vi "Main.vi"() -> ()   [LabVIEW 2017]
doc: "The myRIO Project template acquires acceleration data from the onboard accelerometer and displays the changes of acceleration values in a waveform chart."
uses:
  <vilib>/myRIO/Common/Instrument Driver Framework/myRIO v1.0/Encoder/typedefs/Encoder Count Direction Enum.ctl
  Motor Status Enum.ctl
  <vilib>/myRIO/Instrument Drivers/Onboard IO/PWM/typedefs/PWM Reference.ctl
  <vilib>/myRIO/Common/Instrument Driver Framework/Utilities/typedefs/myRIO Generic Hardware Reference.ctl
  <vilib>/myRIO/Common/Instrument Driver Framework/Utilities/typedefs/Hardware Version Enum.ctl
  <vilib>/myRIO/Common/Instrument Driver Framework/Utilities/typedefs/myRIO v1.0 Reference.ctl
  <vilib>/myRIO/Common/Instrument Driver Framework/Utilities/typedefs/Generic FPGA Reference.ctl
  <vilib>/myRIO/Common/Instrument Driver Framework/myRIO v1.0/PWM/typedefs/PWM Channels Enum.ctl
  <vilib>/myRIO/Instrument Drivers/Onboard IO/PWM/typedefs/PWM Configuration.ctl
  <vilib>/userdefined/High Color/nirio_resource_hc.ctl
  <vilib>/myRIO/Common/Instrument Driver Framework/Utilities/vis/Is FPGA Ref Available.vi
  <vilib>/myRIO/Common/Instrument Driver Framework/myRIO v1.0/PWM/vis/myRIO v1.1 Open PWM.vi
  <vilib>/myRIO/Instrument Drivers/Onboard IO/PWM/vis/Set Duty Cycle and Frequency.vi
  <vilib>/myRIO/Common/Instrument Driver Framework/Utilities/vis/Validate Channels.vi
  <vilib>/myRIO/Common/Instrument Driver Framework/myRIO v1.0/PWM/vis/myRIO v1.0 Reserve PWM.vi
  <vilib>/myRIO/Common/Instrument Driver Framework/myRIO v1.0/UART/vis/myRIO v1.0 Close UART.vi
  <vilib>/myRIO/Common/Instrument Driver Framework/myRIO v1.0/PWM/vis/myRIO v1.0 Build MUX Configuration PWM.vi
  <vilib>/myRIO/Common/Instrument Driver Framework/myRIO v1.0/Resource Manager/vis/myRIO v1.0 Reserve Channel List.vi
  <vilib>/myRIO/Common/Instrument Driver Framework/myRIO v1.0/Resource Manager/vis/myRIO v1.0 Create Configuration List.vi
  <vilib>/myRIO/Common/Instrument Driver Framework/myRIO v1.0/Resource Manager/vis/myRIO v1.0 Reserve Channel.vi
  <vilib>/myRIO/Common/Instrument Driver Framework/myRIO v1.0/Resource Manager/vis/myRIO v1.0 Unreserve Channel.vi
  <vilib>/myRIO/Common/Instrument Driver Framework/myRIO v1.0/Resource Manager/vis/myRIO v1.0 Build Mutex Name.vi
  <vilib>/Utility/VariantDataType/GetNumericInfo.vi
  <vilib>/Utility/error.llb/Error Cluster From Error Code.vi
  <vilib>/myRIO/Common/Instrument Driver Framework/myRIO v1.0/myRIO v1.1 Open.vi
  <vilib>/myRIO/Common/Instrument Driver Framework/Utilities/vis/IO Manager.vi
  <vilib>/myRIO/Common/Instrument Driver Framework/Utilities/vis/Configuration Manager.vi
  <vilib>/myRIO/Common/Instrument Driver Framework/myRIO v1.0/Resource Manager/vis/myRIO v1.0 Configure IO.vi
  <vilib>/myRIO/Common/Instrument Driver Framework/myRIO v1.0/myRIO v1.0 Close.vi
  <vilib>/myRIO/Common/Instrument Driver Framework/myRIO v1.0/PWM/vis/myRIO v1.0 Write PWM.vi
  <vilib>/myRIO/Common/Instrument Driver Framework/Utilities/vis/FPGA Ref Manager.vi
  <vilib>/myRIO/Common/Instrument Driver Framework/myRIO v1.0/myRIO v1.0 Reset FPGA.vi
  <vilib>/myRIO/Common/Instrument Driver Framework/myRIO v1.0/IRQ/vis/myRIO v1.0 IRQ Info FGV.vi
  <vilib>/myRIO/Common/Instrument Driver Framework/myRIO v1.0/IRQ/vis/myRIO v1.0 Timer IRQ Info FGV.vi
  <vilib>/myRIO/Common/Instrument Driver Framework/myRIO v1.0/IRQ/vis/myRIO v1.0 ISR Agent.vi
  <vilib>/myRIO/Express VI/Onboard IO/PWM/PWM Express VI.xnode
  <vilib>/myRIO/Instrument Drivers/Onboard IO/PWM/vis/myRIO PWM Open.xnode
  <vilib>/myRIO/Instrument Drivers/Utilities/Utilities.lvlib
  <vilib>/myRIO/Instrument Drivers/Onboard IO/PWM/PWM.lvlib
panel:
  out "X Axis state":T1
  out "Y Axis state":T1
  out "Loop Runtime (s)":u32
  in  "Clear Chart History":bool
  in  "Coordinates Input":cluster{"X-axis (mm)":dbl, "Y-axis (mm)":dbl}
  out "Y Axis":T2(graph)
  out "X Axis":T2(graph)
  in  "X Axis Motor Target":T3
  out "X Axis Motor Params":T4
  in  "Y Axis Motor Target":T5
  out "Y Axis Motor Params":T5
  in  "stop":bool
  out "Output String":string
  out "Encoder Output":T7
  out "Total Runtime (s)":dbl format="%.2f"
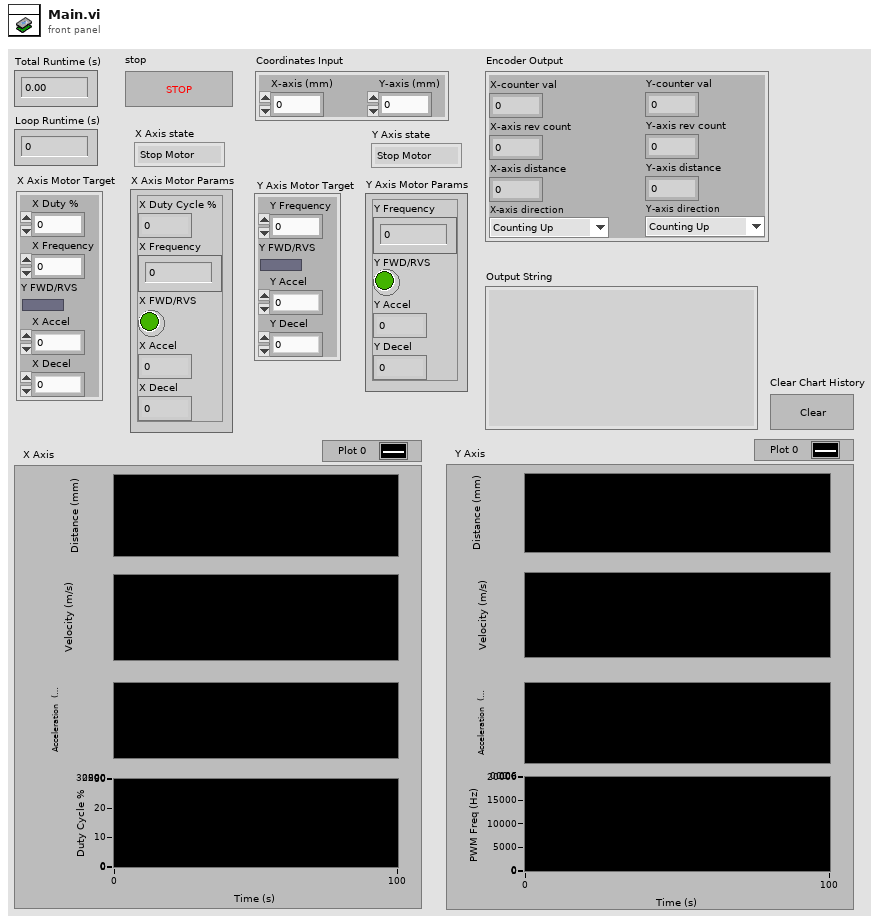
[diagram p1: front panel]
types:
  T1 = typedef "Motor Status Enum.ctl" = enum16{"Stop Motor", "Read Inputs", "Steady Speed", "Accelerate", "Decelerate"}
  T2 = cluster{"X-axis distance":dbl, dbl, dbl, "X Frequency":dbl}
  T3 = cluster{"X Frequency":dbl, "Y FWD/RVS":bool, "X Accel":dbl, "X Decel":dbl, "X Duty %":dbl}
  T4 = cluster{"X Frequency":dbl, "X FWD/RVS":bool, "X Accel":dbl, "X Decel":dbl, "X Duty Cycle %":dbl}
  T5 = cluster{"Y Frequency":dbl, "Y FWD/RVS":bool, "Y Accel":dbl, "Y Decel":dbl}
  T6 = typedef "Encoder Count Direction Enum.ctl" = enum16{"Counting Up", "Counting Down"}
  T7 = cluster{"Y-axis rev count":dbl, "Y-axis distance":dbl, "X-axis rev count":dbl, "X-axis distance":dbl, "Y-axis direction":T6, "X-axis direction":T6, "X-counter val":i32, "Y-counter val":i32}
  T8 = cluster{"X-axis distance":dbl, dbl, dbl, "X Frequency":dbl}[]
  T9 = cluster{dbl, dbl, "X-axis distance":dbl, "X Duty Cycle %":dbl, "X Frequency":dbl, "Y-axis distance":dbl, "Y Frequency":dbl, "X Accel":dbl, "X Decel":dbl, "Y Accel":dbl, "Y Decel":dbl, "X-axis (mm)":dbl, "Y-axis (mm)":dbl}
  T10 = cluster{"X-axis distance":dbl, dbl, dbl, "X Duty Cycle %":dbl}
  T11 = cluster{"Y-axis distance":dbl, dbl, dbl, "Y Frequency":dbl}
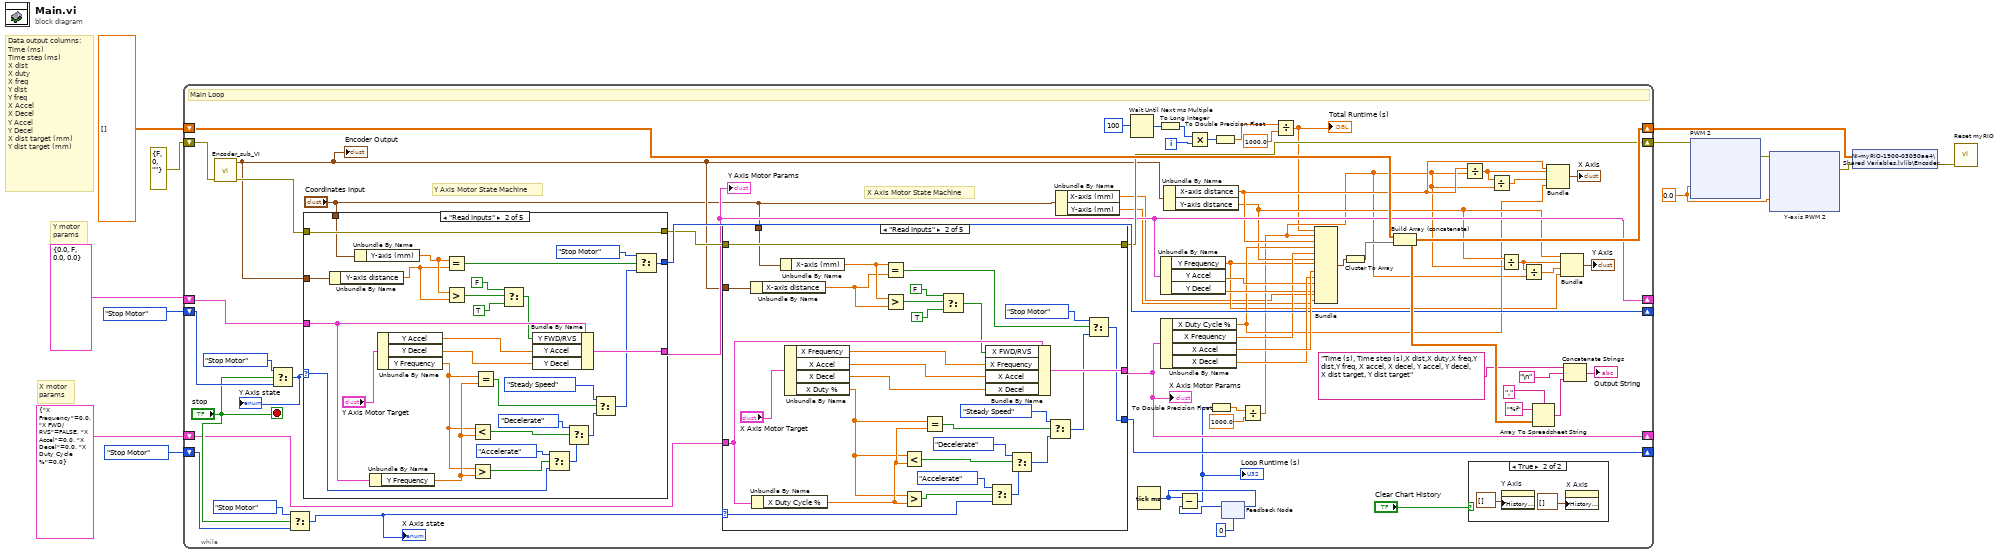
[diagram p0: block diagram]
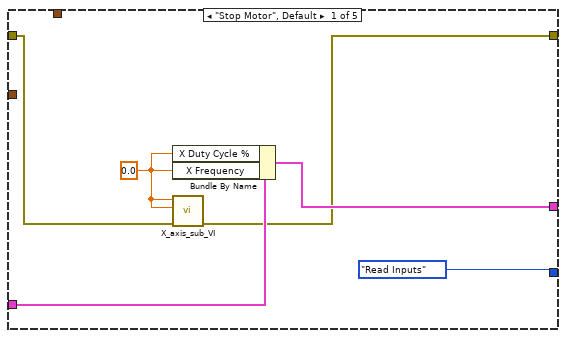
[diagram p3: hidden frame]
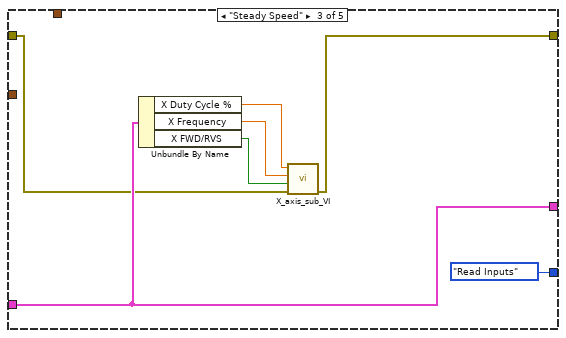
[diagram p4: hidden frame]
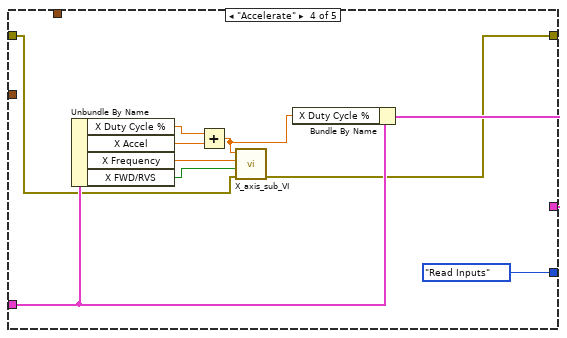
[diagram p5: hidden frame]
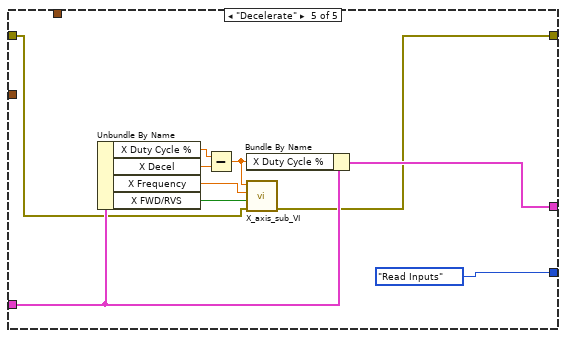
[diagram p6: hidden frame]
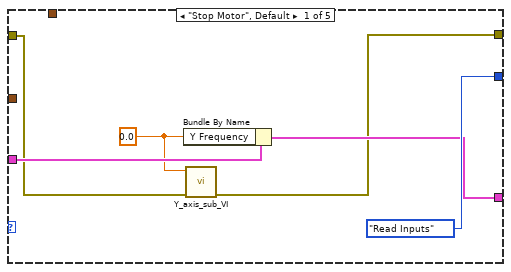
[diagram p7: hidden frame]
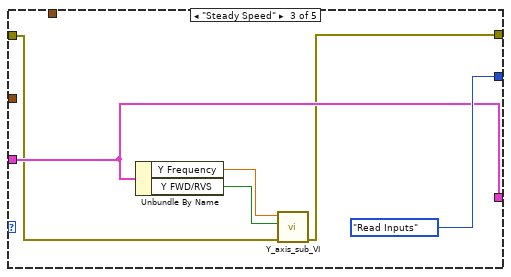
[diagram p8: hidden frame]
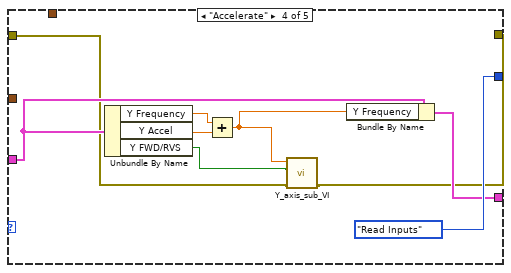
[diagram p9: hidden frame]
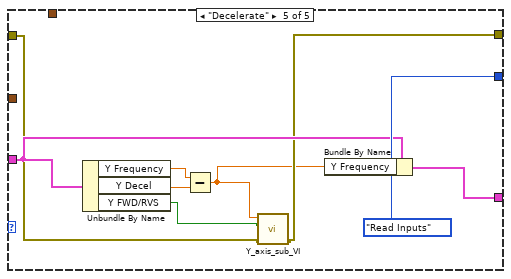
[diagram p10: hidden frame]
diagram:
  w5 = 0.0 ("Frequency [Hz]")
  # "X motor \nparams"
  # "Y motor \nparams"
  # "Data output columns:\nTime (ms)\nTime step (ms)\nX dist\nX duty\nX freq\nY dist\nY freq\nX Accel\nX Decel\nY Accel\nY Decel\nX dist target (mm)\nY dist target (mm)"
  n1 = while {
    shift-right: [w47] -> w12
    shift-left: errorcluster {"status"=FALSE, "code"=0, "source"=""} ("error in (no error)") -> [w74]
    shift-right: [w70] -> w8
    shift-left: dbl[][] [] -> [w69]
    shift-right: [w39] -> _
    shift-left: T5 {"Y Frequency"=0.0, "Y FWD/RVS"=FALSE, "Y Accel"=0.0, "Y Decel"=0.0} ("Y Axis Motor Params 2") -> [w60]
    shift-right: [w59] -> _
    shift-left: Motor_Status_Enum."Stop Motor" -> [w57]
    shift-right: [w50] -> _
    shift-left: Motor_Status_Enum."Stop Motor" -> [w52]
    shift-right: [w40] -> _
    shift-left: T4 {"X Frequency"=0.0, "X FWD/RVS"=FALSE, "X Accel"=0.0, "X Decel"=0.0, "X Duty Cycle %"=0.0} ("X Axis Motor Params 3") -> [w49]
    i -> [w73]
    stop <- "stop" stop-if-true
    # "X Axis Motor State Machine"
    # "Y Axis Motor State Machine"
    # "Main Loop"
    n2 = call "Encoder_sub_VI.vi"("error in (no error)"=w74) -> ("error out"=w55:errorcluster, "Encoder Output"=w38:T7)  [unwired: 9 in]
    "Encoder Output" <- w38
    n3 = Select(t=Motor_Status_Enum."Stop Motor", s="stop", f=w57) -> (s? t:f=w58:T1)
    "Y Axis state" <- w58
    n4 = Select(t=Motor_Status_Enum."Stop Motor", s="stop", f=w52) -> (s? t:f=w53:T1)
    "X Axis state" <- w53
    n5 = case shown="\"Read Inputs\"" w58 {
      selector: w58 -> [_ w160 _ _ _]
      tunnel: w60 -> [w145 w161 w177 w186 w194]
      tunnel: [Motor_Status_Enum."Read Inputs" w152 Motor_Status_Enum."Read Inputs" Motor_Status_Enum."Read Inputs" Motor_Status_Enum."Read Inputs"] -> w59
      tunnel: [w143 w162 w177 w185 w195] -> w39
      tunnel: w55 -> [w141 w159 w176 w182 w192]
      tunnel: [w142 w159 w175 w181 w193] -> w48
      tunnel: w38 -> [_ w158 _ _ _]
      tunnel: "Coordinates Input" -> [_ w146 _ _ _]
      frame "Stop Motor", Default {
        w140 = 0.0 ("Y Frequency")
        n6 = Bundle By Name(cluster=w145, "Y Frequency"=w140) -> (w143:T5)
        n7 = call "Y_axis_sub_VI.vi"("error in (no error)"=w141, "Frequency"=w140) -> ("error out"=w142:errorcluster)  [unwired: 9 in]
      }
      frame "Read Inputs" {
        n8 = Unbundle By Name(w158) -> ("Y-axis distance"=w155:dbl)
        n9 = Unbundle By Name(w146) -> ("Y-axis (mm)"=w156:dbl)
        n10 = Unbundle By Name(w161) -> ("Y Frequency"=w168:dbl)
        n11 = Unbundle By Name("Y Axis Motor Target") -> ("Y Accel"=w172:dbl, "Y Decel"=w173:dbl, "Y Frequency"=w157:dbl)
        n12 = Equal?(x=w156, y=w155) -> (x = y?=w154:bool)
        n13 = Greater?(x=w156, y=w155) -> (0:w150:bool)
        n14 = Less?(x=w157, y=w168) -> (x < y?=w165:bool)
        n15 = Greater?(x=w157, y=w168) -> (0:w174:bool)
        n16 = Equal?(x=w157, y=w168) -> (x = y?=w169:bool)
        n17 = Select(t=FALSE, s=w150, f=TRUE) -> (s? t:f=w147:bool)
        n18 = Bundle By Name(cluster=w161, "Y FWD/RVS"=w147, "Y Accel"=w172, "Y Decel"=w173) -> (w162:T5)
        n19 = Select(t=Motor_Status_Enum."Accelerate", s=w174, f=w160) -> (s? t:f=w167:T1)
        n20 = Select(t=Motor_Status_Enum."Decelerate", s=w165, f=w167) -> (s? t:f=w170:T1)
        n21 = Select(t=Motor_Status_Enum."Steady Speed", s=w169, f=w170) -> (s? t:f=w151:T1)
        n22 = Select(t=Motor_Status_Enum."Stop Motor", s=w154, f=w151) -> (s? t:f=w152:T1)
      }
      frame "Steady Speed" {
        n23 = Unbundle By Name(w177) -> ("Y Frequency"=w179:dbl, "Y FWD/RVS"=w180:bool)
        n24 = call "Y_axis_sub_VI.vi"("error in (no error)"=w176, "FWD/RVS"=w180, "Frequency"=w179) -> ("error out"=w175:errorcluster)  [unwired: 8 in]
      }
      frame "Accelerate" {
        n25 = Unbundle By Name(w186) -> ("Y Frequency"=w188:dbl, "Y Accel"=w189:dbl, "Y FWD/RVS"=w183:bool)
        n26 = Add(x=w188, y=w189) -> (x+y=w184:dbl)
        n27 = call "Y_axis_sub_VI.vi"("error in (no error)"=w182, "FWD/RVS"=w183, "Frequency"=w184) -> ("error out"=w181:errorcluster)  [unwired: 8 in]
        n28 = Bundle By Name(cluster=w186, "Y Frequency"=w184) -> (w185:T5)
      }
      frame "Decelerate" {
        n29 = Unbundle By Name(w194) -> ("Y Frequency"=w198:dbl, "Y Decel"=w197:dbl, "Y FWD/RVS"=w191:bool)
        n30 = Subtract(x=w198, y=w197) -> (x-y=w190:dbl)
        n31 = call "Y_axis_sub_VI.vi"("error in (no error)"=w192, "FWD/RVS"=w191, "Frequency"=w190) -> ("error out"=w193:errorcluster)  [unwired: 8 in]
        n32 = Bundle By Name(cluster=w194, "Y Frequency"=w190) -> (w195:T5)
      }
    }
    "Y Axis Motor Params" <- w39
    n33 = case shown="\"Read Inputs\"" w53 {
      selector: w53 -> [_ w100 _ _ _]
      tunnel: [Motor_Status_Enum."Read Inputs" w84 Motor_Status_Enum."Read Inputs" Motor_Status_Enum."Read Inputs" Motor_Status_Enum."Read Inputs"] -> w50
      tunnel: [w79 w99 w116 w123 w133] -> w40
      tunnel: w49 -> [w80 w98 w116 w122 w132]
      tunnel: w48 -> [w78 w96 w114 w121 w131]
      tunnel: [w77 w96 w113 w120 w130] -> w47
      tunnel: w38 -> [_ w94 _ _ _]
      tunnel: "Coordinates Input" -> [_ w83 _ _ _]
      frame "Stop Motor", Default {
        w82 = 0.0 ("Y Frequency")
        n34 = Bundle By Name(cluster=w80, "X Duty Cycle %"=w82, "X Frequency"=w82) -> (w79:T4)
        n35 = call "X_axis_sub_VI.vi"("error in (no error)"=w78, "Frequency"=w82, "Duty Cycle %"=w82) -> ("error out"=w77:errorcluster)  [unwired: 8 in]
      }
      frame "Read Inputs" {
        n36 = Unbundle By Name(w94) -> ("X-axis distance"=w89:dbl)
        n37 = Unbundle By Name(w98) -> ("X Duty Cycle %"=w111:dbl)
        n38 = Unbundle By Name(w83) -> ("X-axis (mm)"=w90:dbl)
        n39 = Unbundle By Name("X Axis Motor Target") -> ("X Frequency"=w103:dbl, "X Accel"=w101:dbl, "X Decel"=w102:dbl, "X Duty %"=w95:dbl)
        n40 = Equal?(x=w90, y=w89) -> (x = y?=w88:bool)
        n41 = Greater?(x=w90, y=w89) -> (0:w92:bool)
        n42 = Less?(x=w95, y=w111) -> (x < y?=w106:bool)
        n43 = Greater?(x=w95, y=w111) -> (0:w104:bool)
        n44 = Equal?(x=w95, y=w111) -> (x = y?=w110:bool)
        n45 = Select(t=FALSE, s=w92, f=TRUE) -> (s? t:f=w85:bool)
        n46 = Bundle By Name(cluster=w98, "X FWD/RVS"=w85, "X Frequency"=w103, "X Accel"=w101, "X Decel"=w102) -> (w99:T4)
        n47 = Select(t=Motor_Status_Enum."Accelerate", s=w104, f=w100) -> (s? t:f=w108:T1)
        n48 = Select(t=Motor_Status_Enum."Decelerate", s=w106, f=w108) -> (s? t:f=w109:T1)
        n49 = Select(t=Motor_Status_Enum."Steady Speed", s=w110, f=w109) -> (s? t:f=w86:T1)
        n50 = Select(t=Motor_Status_Enum."Stop Motor", s=w88, f=w86) -> (s? t:f=w84:T1)
      }
      frame "Steady Speed" {
        n51 = Unbundle By Name(w116) -> ("X Duty Cycle %"=w118:dbl, "X Frequency"=w117:dbl, "X FWD/RVS"=w119:bool)
        n52 = call "X_axis_sub_VI.vi"("error in (no error)"=w114, "FWD/RVS"=w119, "Frequency"=w117, "Duty Cycle %"=w118) -> ("error out"=w113:errorcluster)  [unwired: 7 in]
      }
      frame "Accelerate" {
        n53 = Unbundle By Name(w122) -> ("X Duty Cycle %"=w125:dbl, "X Accel"=w126:dbl, "X Frequency"=w127:dbl, "X FWD/RVS"=w129:bool)
        n54 = Add(x=w125, y=w126) -> (x+y=w128:dbl)
        n55 = call "X_axis_sub_VI.vi"("error in (no error)"=w121, "FWD/RVS"=w129, "Frequency"=w127, "Duty Cycle %"=w128) -> ("error out"=w120:errorcluster)  [unwired: 7 in]
        n56 = Bundle By Name(cluster=w122, "X Duty Cycle %"=w128) -> (w123:T4)
      }
      frame "Decelerate" {
        n57 = Unbundle By Name(w132) -> ("X Duty Cycle %"=w135:dbl, "X Decel"=w136:dbl, "X Frequency"=w137:dbl, "X FWD/RVS"=w139:bool)
        n58 = Subtract(x=w135, y=w136) -> (x-y=w138:dbl)
        n59 = Bundle By Name(cluster=w132, "X Duty Cycle %"=w138) -> (w133:T4)
        n60 = call "X_axis_sub_VI.vi"("error in (no error)"=w131, "FWD/RVS"=w139, "Frequency"=w137, "Duty Cycle %"=w138) -> ("error out"=w130:errorcluster)  [unwired: 7 in]
      }
    }
    "X Axis Motor Params" <- w40
    n61 = Unbundle By Name("Coordinates Input") -> ("X-axis (mm)"=w15:dbl, "Y-axis (mm)"=w14:dbl)
    n62 = Wait Until Next ms Multiple(millisecond multiple=u32 100 ("milliseconds to wait")) -> (millisecond timer value=w61:u32)
    n63 = Tick Count (ms)() -> (millisecond timer value=w23:u32)
    n64 = To Long Integer(number=w61) -> (32bit integer=w64:i32)
    n65 = Unbundle By Name(w39) -> ("Y Frequency"=w27:dbl, "Y Accel"=w66:dbl, "Y Decel"=w65:dbl)
    n66 = Unbundle By Name(w40) -> ("X Duty Cycle %"=w28:dbl, "X Frequency"=w33:dbl, "X Accel"=w68:dbl, "X Decel"=w67:dbl)
    n67 = Unbundle By Name(w38) -> ("X-axis distance"=w37:dbl, "Y-axis distance"=w31:dbl)
    n68 = Multiply(x=w64, y=w73) -> (x*y=w62:i32)
    n69 = To Double Precision Float(number=w62) -> (double precision float=w17:dbl)
    n70 = feedback-in #1(w23) -> ()
    n71 = feedback #1(u32 0) -> (w24:u32)
    n72 = Subtract(x=w23, y=w24) -> (x-y=w22:u32)
    "Loop Runtime (s)" <- w22
    n73 = To Double Precision Float(number=w22) -> (double precision float=w20:dbl)
    n74 = Divide(x=w20, y=1000.0) -> (x/y=w19:dbl)
    n75 = Divide(x=w17, y=1000.0) -> (x/y=w13:dbl)
    "Total Runtime (s)" <- w13
    n76 = Bundle(w13, w19, "X-axis distance"=w37, "X Duty Cycle %"=w28, "X Frequency"=w33, "Y-axis distance"=w31, "Y Frequency"=w27, "X Accel"=w68, "X Decel"=w67, "Y Accel"=w66, "Y Decel"=w65, "X-axis (mm)"=w15, "Y-axis (mm)"=w14) -> (w71:T9)  [unwired: 1 in]
    n77 = Cluster To Array(cluster=w71) -> (array=w72:dbl[])
    n78 = Build Array (concatenate)(w69, w72) -> (w70:dbl[][])
    n79 = Divide(x=w37, y=w19) -> (x/y=w36:dbl)
    n80 = case shown="True" "Clear Chart History" {
      frame False {
      }
      frame True {
        n81 = property on="Y Axis" class="WFChart (strict)"("History Data"=T8 []) -> ()  [unwired: 2 in, 2 out]
        n82 = property on="X Axis" class="WFChart (strict)"("History Data"=T8 []) -> ()  [unwired: 2 in, 2 out]
      }
    }
    n83 = Divide(x=w36, y=w19) -> (x/y=w35:dbl)
    n84 = Divide(x=w31, y=w19) -> (x/y=w30:dbl)
    n85 = Divide(x=w30, y=w19) -> (x/y=w29:dbl)
    n86 = Array To Spreadsheet String(delimiter (Tab)=",", array=w70, 3:"%f" ("format string")) -> (spreadsheet string=w45:string)
    n87 = Bundle("X-axis distance"=w37, w36, w35, "X Duty Cycle %"=w28) -> (→"X Axis":T10)  [unwired: 1 in]
    n88 = Bundle("Y-axis distance"=w31, w30, w29, "Y Frequency"=w27) -> (→"Y Axis":T11)  [unwired: 1 in]
    n89 = Concatenate Strings("Time (s), Time step (s),X dist,X duty,X freq,Y dist,Y freq, X accel, X decel, Y accel, Y decel, X dist target, Y dist target", "\n", w45) -> (→"Output String":string)
  }
  n90 = xnode "PWM 2"("Frequency [Hz]"=w5, "error in (no error)"=w12) -> ("error out"=w7:errorcluster)
  n91 = xnode "Y-axis PWM 2"("Frequency [Hz]"=w5, "error in (no error)"=w7) -> ("error out"=w6:errorcluster)
  n92 = shared-variable "NI-myRIO-1900-03050ae4\\Shared Variables.lvlib\\Encoder Data"(w8, error in=w6) -> (error out=w9:errorcluster)
  n93 = call <vilib>:"Reset myRIO.vi"("error in (no error)"=w9) -> ()  [unwired: 10 in, 1 out]
